vi "CanChannelSendMsg.vi"(4 "error in":errorcluster {"code" format="%.0x"}, 5 "CAN message":T1 {"DLC" max=8; "Type" items=["data"]; "Data"."[4]" format="%02x"; "Data"."[7]" format="%02x"; "Data"."[6]" format="%02x"; "Data"."[5]" format="%02x"; "Data"."[3]" format="%02x"; "Data"."[2]" format="%02x"; "Data"."[1]" format="%02x"; "Data"."[0]" format="%02x"; "Arbitration ID" format="%08x"; "Timestamp" format="%08x"}, 6 "Milliseconds":u32 format="%x", 7 "CAN Channel Handle in":u32 format="%x") -> (0 "error out":errorcluster {"code" format="%.0x"}, 2 "Send OK":bool, 3 "CAN Channel Handle out":u32)   [LabVIEW 2011]
doc: "Places the CAN message in the transmit FIFO of the channel. The VI waits until the message is placed in the transmit FIFO, but does not wait for the message to be transmitted over the CAN bus."
uses:
  vcilva.dll
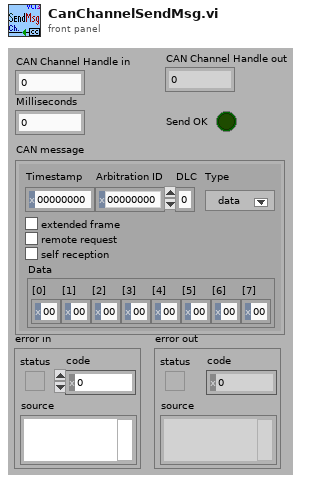
[diagram p1: front panel]
types:
  T1 = cluster{"Timestamp":u32, "Arbitration ID":u32, "DLC":u8, "Type":u8, "extended frame":bool, "remote request":bool, "self reception":bool, "Data":cluster{"[0]":u8, "[1]":u8, "[2]":u8, "[3]":u8, "[4]":u8, "[5]":u8, "[6]":u8, "[7]":u8}}
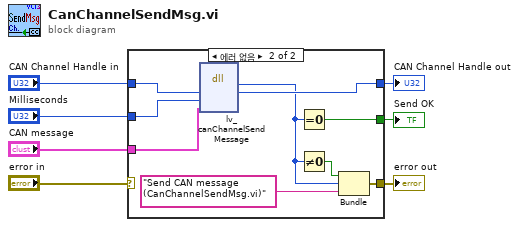
[diagram p0: block diagram]
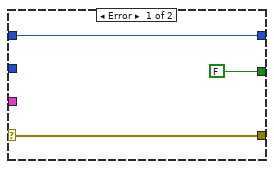
[diagram p2: hidden frame]
diagram:
  n1 = case shown="에러 없음" "error in" {
    selector: "error in" -> [w10 _]
    tunnel: [w10 w19] -> w7
    tunnel: "CAN Channel Handle in" -> [w9 w16]
    tunnel: [w9 w15] -> w5
    tunnel: "CAN message" -> [_ w14]
    tunnel: "Milliseconds" -> [_ w13]
    tunnel: [FALSE w11] -> w1
    frame Error {
    }
    frame No Error {
      n2 = dll-call lib="vcilva.dll" fn="lv_canChannelSendMessage"("hCanChn"=w16, "dwMilliseconds"=w13, "CAN message"=w14) -> (w12:i32, "hCanChn"=w15:u32)  [unwired: 5 in, 2 out]
      n3 = Equal To 0?(x=w12) -> (x = 0?=w11:bool)
      n4 = Not Equal To 0?(x=w12) -> (x != 0?=w18:bool)
      n5 = Bundle(w18, w12, "Send CAN message (CanChannelSendMsg.vi)") -> (w19:errorcluster)  [unwired: 1 in]
    }
  }
  "error out" <- w7
  "CAN Channel Handle out" <- w5
  "Send OK" <- w1
